vi "sir_v5.vi"() -> ()   [LabVIEW 2009]
panel:
  out "Sirul sirul din spate":string="Electrica"
  out "Sirul cautat":string="Inginerie "
  in  "Sirul 2":string="Inginerie "
  out "Pozitia dupa sirului cautat":dbl=21.0
  in  "stop":bool
  out "Sirul din fata":string="Catedra de "
  in  "Sirul 1":string="Catedra de Inginerie Electrica"
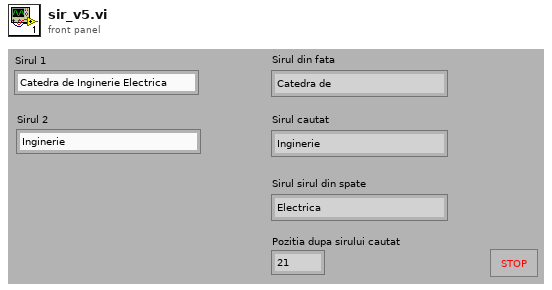
[diagram p1: front panel]
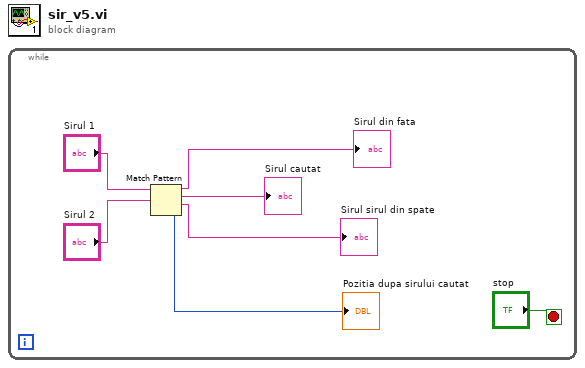
[diagram p0: block diagram]
diagram:
  n1 = while {
    stop <- "stop" stop-if-true
    n2 = Match Pattern(string="Sirul 1", regular expression="Sirul 2") -> (before substring=→"Sirul din fata":string, match substring=→"Sirul cautat":string, after substring=→"Sirul sirul din spate":string, offset past match=→"Pozitia dupa sirului cautat":i32)  [unwired: 1 in]
  }
